vi "Autosampler Move To.vi"(7 "Correlation ID":u32, 8 "error in (no error)":errorcluster, 9 "Index":u16, 10 "Area":enum16{"Home", "Well", "Wash Port"}(ring), 11 "Application in":refnum<class "Application.lvclass">) -> (0 "error out":errorcluster, 3 "Application out":refnum<class "Application.lvclass">)   [LabVIEW 2023, in "Application.lvlib" / "Application.lvclass"]
uses:
  Application.lvclass
  Application.lvclass/Application.ctl
  Hardware/Device Messages/Save CorrID Msg/Save CorrID Msg.lvclass/Save CorrID Msg.ctl
  <vilib>/ActorFramework/Message Enqueuer/Message Enqueuer.lvclass/Message Enqueuer.ctl
  Hardware/Autosampler Messages/Move To Msg/Move To Msg.lvclass/Move To Msg.ctl
  <vilib>/ActorFramework/Message Enqueuer/Enqueue.vi
  Hardware/Device Messages/Save CorrID Msg/Save CorrID Msg.lvclass
  Hardware/Autosampler Messages/Move To Msg/Move To Msg.lvclass
  <vilib>/ActorFramework/Message Priority Queue/Priority Enqueue.vi
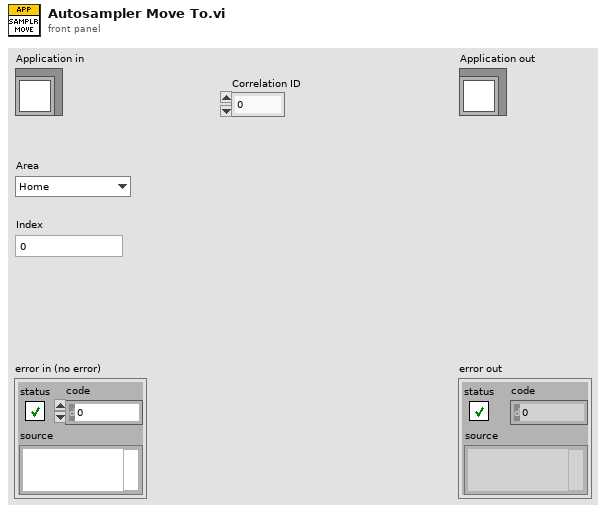
[diagram p1: front panel]
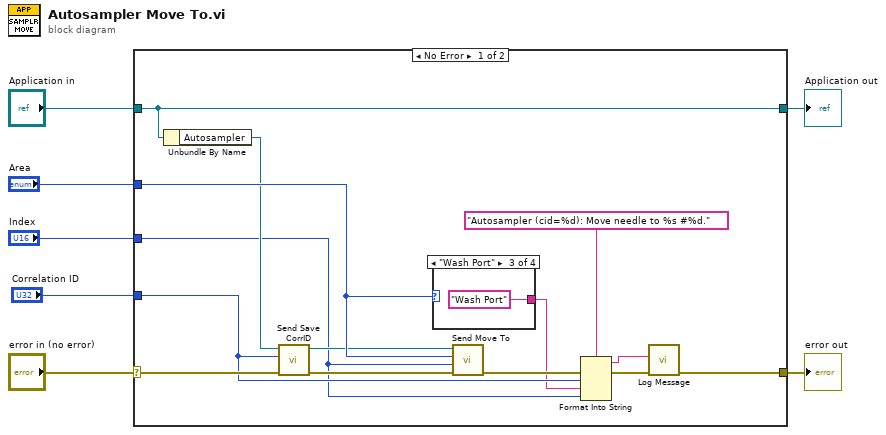
[diagram p0: block diagram]
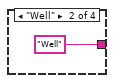
[diagram p3: hidden frame]
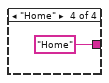
[diagram p4: hidden frame]
diagram:
  n1 = case shown="No Error" "error in (no error)" {
    selector: "error in (no error)" -> [w14 w26]
    tunnel: [w17 w26] -> w6
    tunnel: [w21 w25] -> w4
    tunnel: "Application in" -> [w21 w25]
    tunnel: "Area" -> [w15 _]
    tunnel: "Index" -> [w8 _]
    tunnel: "Correlation ID" -> [w10 _]
    frame No Error {
      n2 = Unbundle By Name(w21) -> ("Autosampler"=w13:refnum<class "Message Enqueuer.lvclass">)
      n3 = call "Send Save CorrID.vi"("error in (no error)"=w14, "Correlation ID"=w10, "Message Enqueuer"=w13) -> ("error out"=w12:errorcluster, "Message Enqueuer out"=w11:refnum<class "Message Enqueuer.lvclass">)  [unwired: 7 in]
      n4 = case shown="\"Wash Port\"" w15 {
        tunnel: [_ "Well" "Wash Port" "Home"] -> w9
        frame Default {
        }
        frame "Well" {
        }
        frame "Wash Port" {
        }
        frame "Home" {
        }
      }
      n5 = call "Send Move To.vi"("error in (no error)"=w12, "Index"=w8, "Area"=w15, "Message Enqueuer"=w11) -> ("error out"=w18:errorcluster)  [unwired: 6 in, 1 out]
      n6 = Format Into String(format string="Autosampler (cid=%d): Move needle to %s #%d.", error in=w18, w10, w9, w8) -> (resulting string=w20:string, error out=w19:errorcluster)  [unwired: 1 in]
      n7 = call "Log Message.vi"("error constant"=w19, "input"=w20) -> ("error constant 2"=w17:errorcluster)  [unwired: 8 in, 1 out]
    }
    frame Error {
    }
  }
  "error out" <- w6
  "Application out" <- w4
